vi "ScaleSimulatedData.vi"(10 "Config":T1={"Max"={"Enable"=TRUE, "New Max Temp"=100.0, "KeepMin"=FALSE}, "Noise"={"Randomize"=TRUE, "Max delta"=0.5}, "Hotspot"={"hotspot"=FALSE, "Rectangle"={"left"=100, "top"=200, "right"=150, "bottom"=250}, "Temperature"=100.0}}, 11 "data in":sgl[][](array[numeric])) -> (3 "data out":sgl[][](array[numeric]))   [LabVIEW 2017, in "IrAcquisition.lvlib"]
uses:
  <vilib>/addons/InsightCM/Devices/Shared/Ir/IrAcquisition/IrAcquisition.lvlib
  <vilib>/addons/InsightCM/Devices/Shared/Ir/IrAcquisition/controls/simScaleConfig.ctl
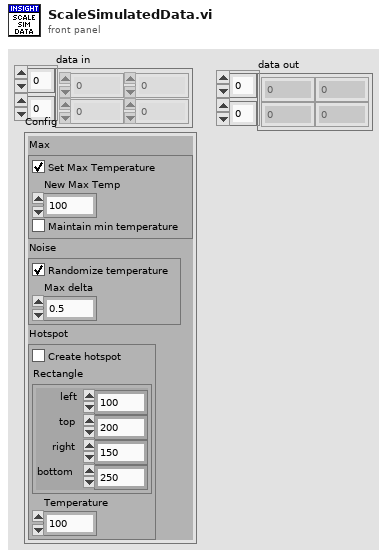
[diagram p1: front panel]
types:
  T1 = typedef "IrAcquisition.lvlib/simScaleConfig.ctl" = cluster{"Max":cluster{"Enable":bool, "New Max Temp":sgl, "KeepMin":bool}, "Noise":cluster{"Randomize":bool, "Max delta":sgl}, "Hotspot":cluster{"hotspot":bool, "Rectangle":cluster{"left":i16, "top":i16, "right":i16, "bottom":i16}, "Temperature":sgl}}
  T2 = cluster{"hotspot":bool, "Rectangle":cluster{"left":i16, "top":i16, "right":i16, "bottom":i16}, "Temperature":sgl}
  T3 = cluster{"left":i16, "top":i16, "right":i16, "bottom":i16}
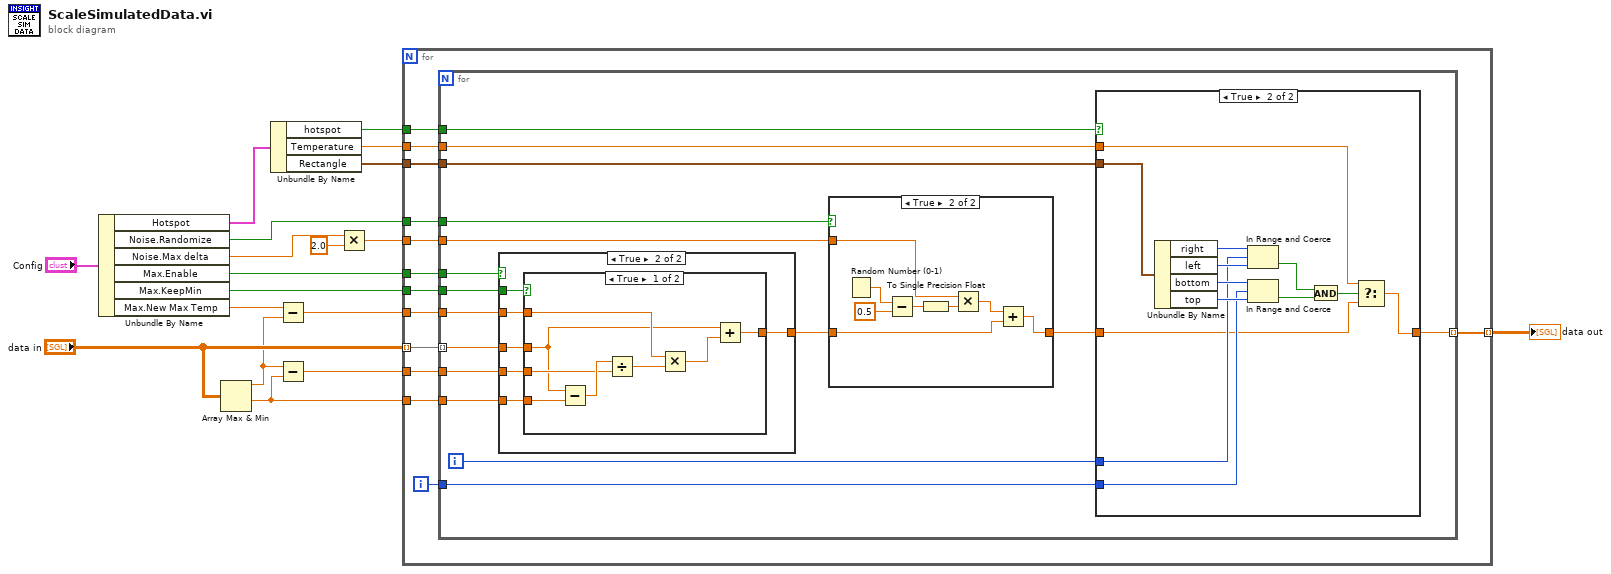
[diagram p0: block diagram]
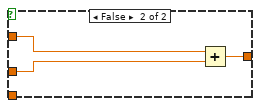
[diagram p3: hidden frame]
diagram:
  n1 = Unbundle By Name("Config") -> ("Hotspot"=w5:T2, "Noise.Randomize"=w6:bool, "Noise.Max delta"=w7:sgl, "Max.Enable"=w1:bool, "Max.KeepMin"=w8:bool, "Max.New Max Temp"=w9:sgl)
  n2 = Array Max & Min(array="data in") -> (max value=w13:sgl, min value=w16:sgl)  [unwired: 2 out]
  n3 = Unbundle By Name(w5) -> ("hotspot"=w4:bool, "Temperature"=w3:sgl, "Rectangle"=w2:T3)
  n4 = Subtract(x=w9, y=w13) -> (x-y=w15:sgl)
  n5 = Subtract(x=w13, y=w16) -> (x-y=w17:sgl)
  n6 = Multiply(x=w7, y=sgl 2.0) -> (x*y=w11:sgl)
  n7 = for {
    tunnel: "data in" -> [w31] mode=indexing
    tunnel: w17 -> [w30]
    tunnel: w16 -> [w29]
    tunnel: w15 -> [w28]
    tunnel: [w27] -> w14 mode=indexing
    tunnel: w8 -> [w26]
    tunnel: w11 -> [w25]
    tunnel: w6 -> [w24]
    tunnel: w2 -> [w23]
    tunnel: w3 -> [w21]
    tunnel: w4 -> [w20]
    tunnel: w1 -> [w19]
    i -> [w22]
    n8 = for {
      tunnel: w31 -> [w44] mode=indexing
      tunnel: w29 -> [w47]
      tunnel: w30 -> [w46]
      tunnel: w28 -> [w45]
      tunnel: [w33] -> w27 mode=indexing
      tunnel: w26 -> [w43]
      tunnel: w25 -> [w42]
      tunnel: w24 -> [w40]
      tunnel: w23 -> [w39]
      tunnel: w22 -> [w37]
      tunnel: w21 -> [w35]
      tunnel: w20 -> [w34]
      tunnel: w19 -> [w32]
      i -> [w38]
      n9 = case shown="True" w32 {
        tunnel: w47 -> [_ w54]
        tunnel: w46 -> [_ w53]
        tunnel: w45 -> [_ w52]
        tunnel: w44 -> [w48 w51]
        tunnel: w43 -> [_ w50]
        tunnel: [w48 w49] -> w41
        frame False {
        }
        frame True {
          n10 = case shown="True" w50 {
            tunnel: w54 -> [w62 _]
            tunnel: w53 -> [w60 _]
            tunnel: w52 -> [w59 w63]
            tunnel: w51 -> [w58 w65]
            tunnel: [w57 w64] -> w49
            frame True {
              n11 = Subtract(x=w58, y=w62) -> (x-y=w61:sgl)
              n12 = Divide(x=w61, y=w60) -> (x/y=w56:sgl)
              n13 = Multiply(x=w59, y=w56) -> (x*y=w55:sgl)
              n14 = Add(x=w58, y=w55) -> (x+y=w57:sgl)
            }
            frame False {
              n15 = Add(x=w63, y=w65) -> (x+y=w64:sgl)
            }
          }
        }
      }
      n16 = case shown="True" w40 {
        tunnel: w42 -> [_ w85]
        tunnel: w41 -> [w80 w83]
        tunnel: [w80 w82] -> w36
        frame False {
        }
        frame True {
          n17 = Random Number (0-1)() -> (number: 0 to 1=w88:dbl)
          n18 = Subtract(x=w88, y=0.5) -> (x-y=w86:dbl)
          n19 = To Single Precision Float(number=w86) -> (single precision float=w81:sgl)
          n20 = Multiply(x=w85, y=w81) -> (x*y=w84:sgl)
          n21 = Add(x=w84, y=w83) -> (x+y=w82:sgl)
        }
      }
      n22 = case shown="True" w34 {
        tunnel: w39 -> [_ w79]
        tunnel: w38 -> [_ w72]
        tunnel: w37 -> [_ w71]
        tunnel: w36 -> [w66 w69]
        tunnel: w35 -> [_ w68]
        tunnel: [w66 w67] -> w33
        frame False {
        }
        frame True {
          n23 = Unbundle By Name(w79) -> ("right"=w78:i16, "left"=w77:i16, "bottom"=w76:i16, "top"=w75:i16)
          n24 = In Range and Coerce(upper limit=w78, x=w72, lower limit=w77) -> (In Range?=w74:bool)  [unwired: 1 out]
          n25 = In Range and Coerce(upper limit=w76, x=w71, lower limit=w75) -> (In Range?=w73:bool)  [unwired: 1 out]
          n26 = And(x=w74, y=w73) -> (x .and. y?=w70:bool)
          n27 = Select(t=w68, s=w70, f=w69) -> (s? t:f=w67:sgl)
        }
      }
    }
  }
  "data out" <- w14
